vi "Digital Serial Acq Cfg Popup.vi"(8 "error in (no error)":errorcluster, 11 "config file in":path caption="Configuration File") -> (0 "error out":errorcluster, 2 "digital serial input settings":T2={"number of channels"=0, "data justification"=enum."Left Justified", "endianness"=enum."LSB First", "channel length"=0, "bit depth"=0, "frame clock rate"=0.0, "bit clock edge sync"=enum."Falling", "master clock source"=enum."Internal", "master clock rate"=2.0, "Logic Level"=enum."3.3 V", "frame sync edge for channel 0"=enum."Rising", "Channel 0 Offset"=0}, 3 "config file out":path caption="Configuration File")   [LabVIEW 2022 SP3, in "Config Dialog.lvlib"]
uses:
  Config Dialog.lvlib
  controls/digital serial audio/digital serial input settings.ctl
  <vilib>/PDM Acquisition Toolkit/shared/controls/PCM Data Justification.ctl
  <vilib>/PDM Acquisition Toolkit/shared/controls/PCM Bit Endianness.ctl
  <vilib>/PDM Acquisition Toolkit/shared/controls/Digital Edge.ctl
  controls/master clock source.ctl
  <vilib>/PDM Acquisition Toolkit/host/Classes/Session/Controls/Logic Levels.ctl
  <vilib>/Utility/miscctls.llb/LVPointTypeDef.ctl
  <vilib>/PDM Acquisition Toolkit/shared/PDM Shared.lvlib
  <vilib>/PDM Acquisition Toolkit/host/Classes/Session/DecoderSession.lvclass
  input configuration file/input cfg file.lvlib
  input configuration file/digital serial/digital serial input cfg file.lvlib
panel:
  in  "master clock source":T1 caption="Master clock source"
  in  "channel 0 offset":u32=1
  in  "Save":bool
  in  "logic level":enum32{"3.3 V", "1.8 V", "1.2 V"}(ring) caption="Logic level"
  in  "master clock rate":dbl=12288000.0 caption="Master clock rate" format="%#_6pHz"
  out "Bit clock rate":dbl=3072000.0 format="%#_6pHz"
  in  "number of channels":u32=2 caption="Number of channels"
  in  "TDM":bool
  in  "RJ":bool
  in  "LJ":bool
  in  "I2S":bool
  in  "bit clock edge sync":enum32{"Rising", "Falling"}(ring)=enum."Falling" caption="Bit clock edge sync"
  in  "frame clock rate":dbl=48000.0 caption="Frame clock rate" format="%#_6pHz"
  in  "data justification":enum32{"Left Justified", "Right Justified"}(ring) caption="Data justification"
  in  "endianness":enum32{"MSB First", "LSB First"}(ring) caption="Endianness"
  in  "bit depth":u32=24 caption="Bit depth"
  in  "channel length":u32=32 caption="Channel length"
  in  "frame sync edge for channel 0":enum32{"Rising", "Falling"}(ring)=enum."Falling" caption="Frame sync edge for Channel 0"
  # "Audio Protocol"
  # "Clock Settings"
  # "Signal Level"
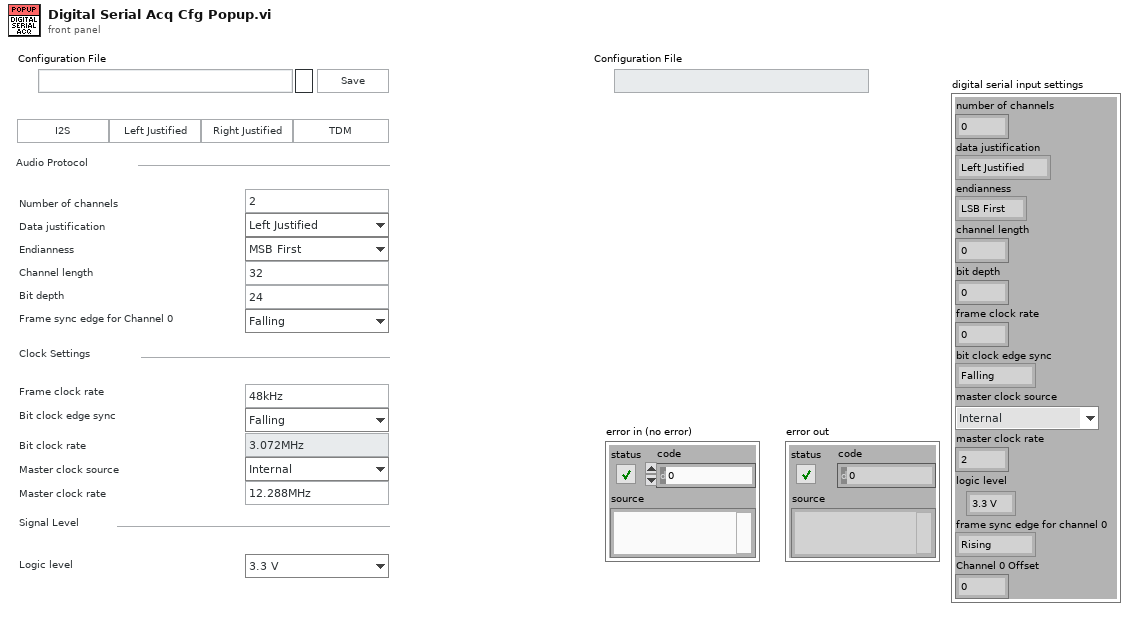
[diagram p1: front panel]
types:
  T1 = typedef "master clock source.ctl" = enum32{"Internal", "External"}
  T2 = typedef "digital serial input settings.ctl" = cluster{"number of channels":u32, "data justification":T3, "endianness":T4, "channel length":u32, "bit depth":u32, "frame clock rate":dbl, "bit clock edge sync":T5, "master clock source":T1, "master clock rate":dbl, "Logic Level":T6, "frame sync edge for channel 0":T5, "Channel 0 Offset":u32}
  T3 = typedef "PDM Shared.lvlib/PCM Data Justification.ctl" = enum16{"Left Justified", "Right Justified"}
  T4 = typedef "PDM Shared.lvlib/PCM Bit Endianness.ctl" = enum16{"MSB First", "LSB First"}
  T5 = typedef "PDM Shared.lvlib/Digital Edge.ctl" = enum8{"Rising", "Falling"}
  T6 = typedef "PDM Acquisition Class Library.lvlib/DecoderSession.lvclass/Logic Levels.ctl" = enum16{"3.3 V", "1.8 V", "1.2 V"}
  T7 = typedef "LVPointTypeDef.ctl" = cluster{"Horizontal":i16, "Vertical":i16}
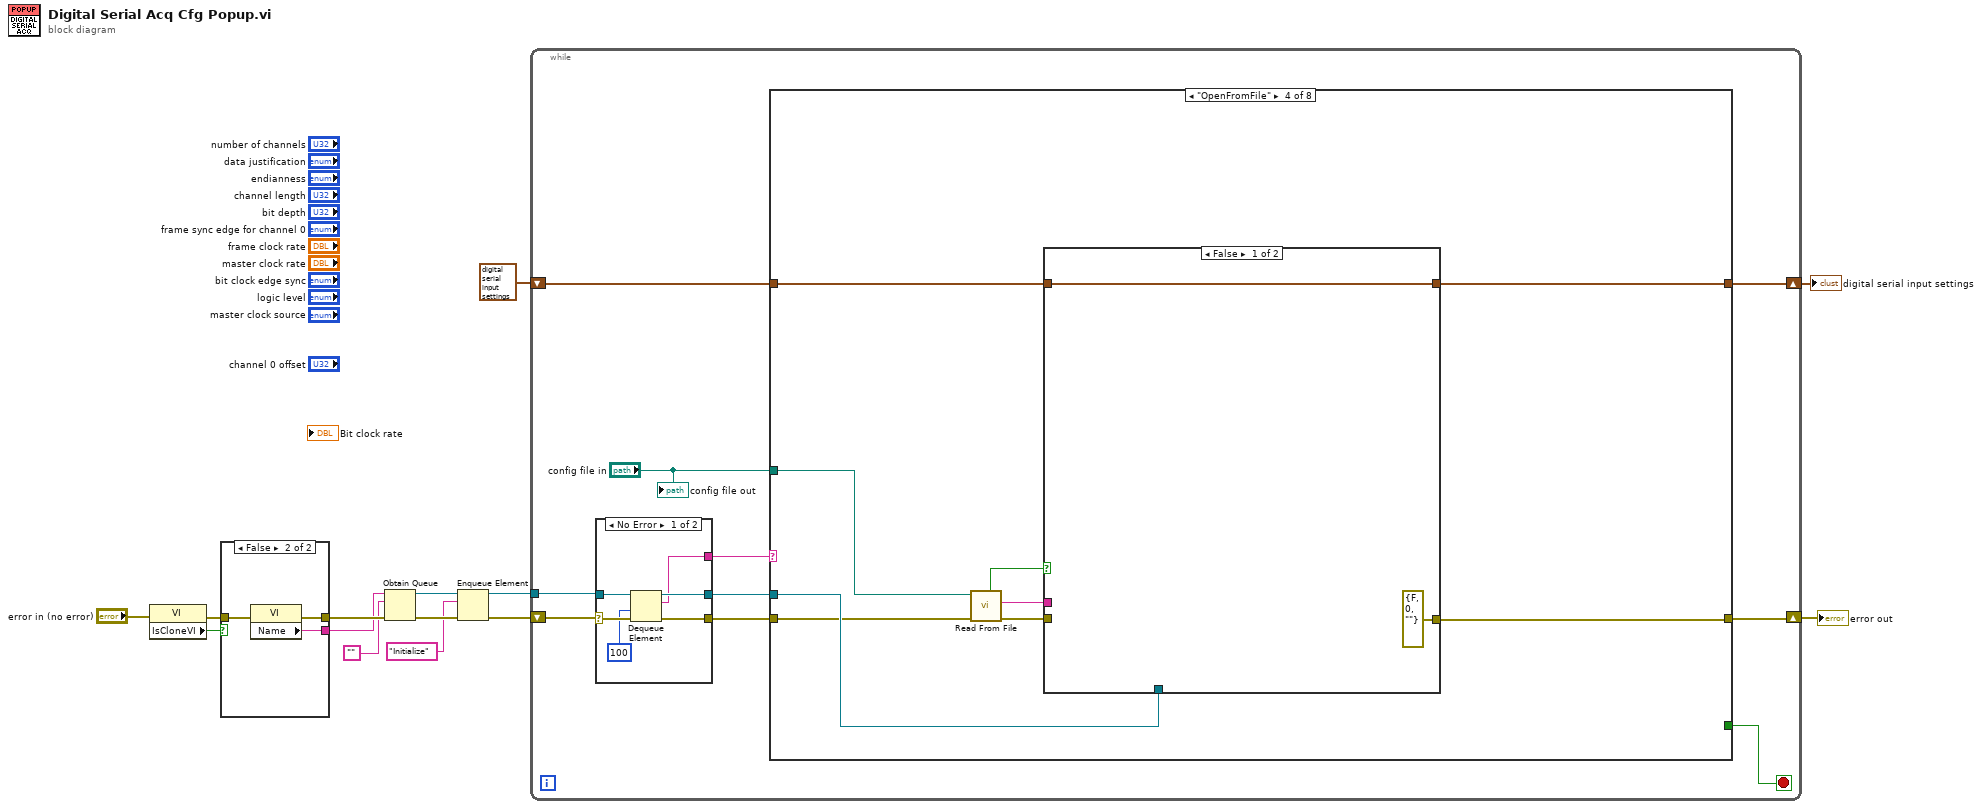
[diagram p0: block diagram]
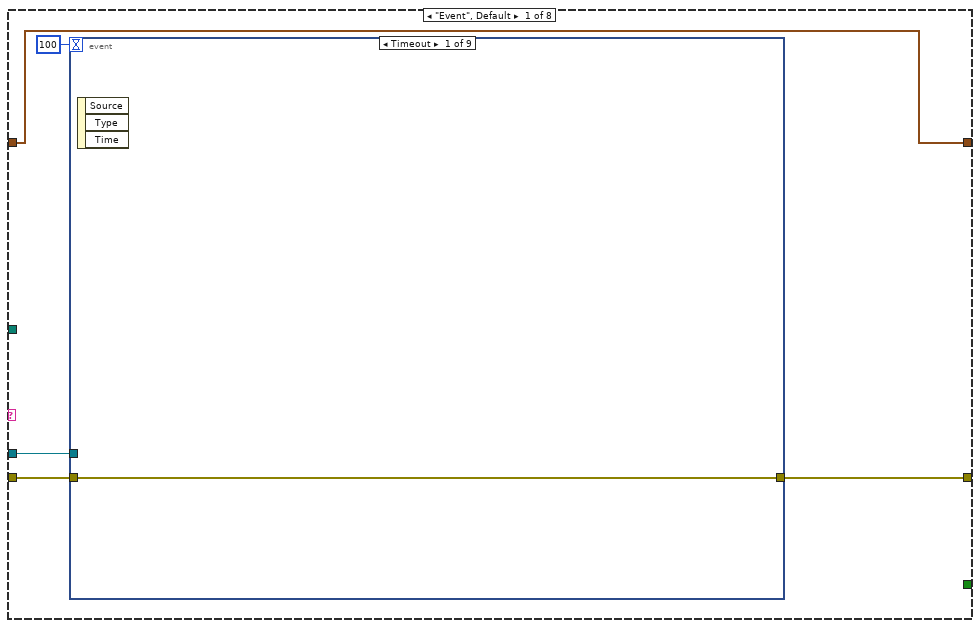
[diagram p2: hidden frame]
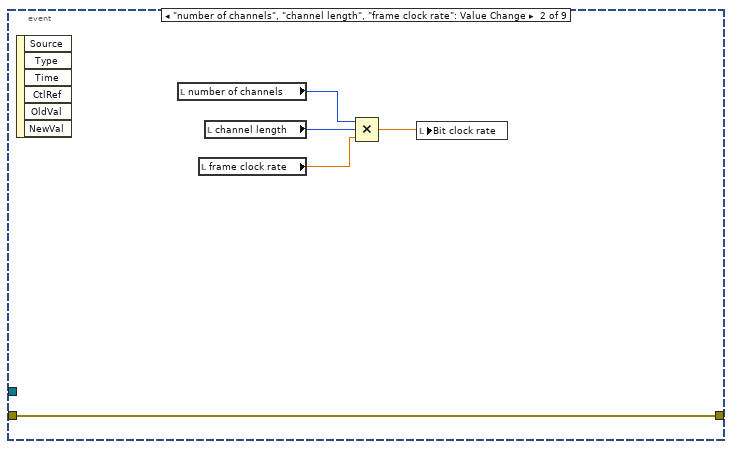
[diagram p3: hidden frame]
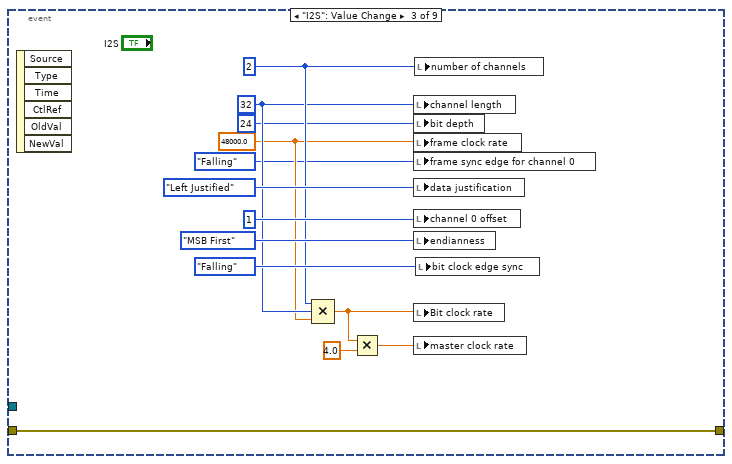
[diagram p4: hidden frame]
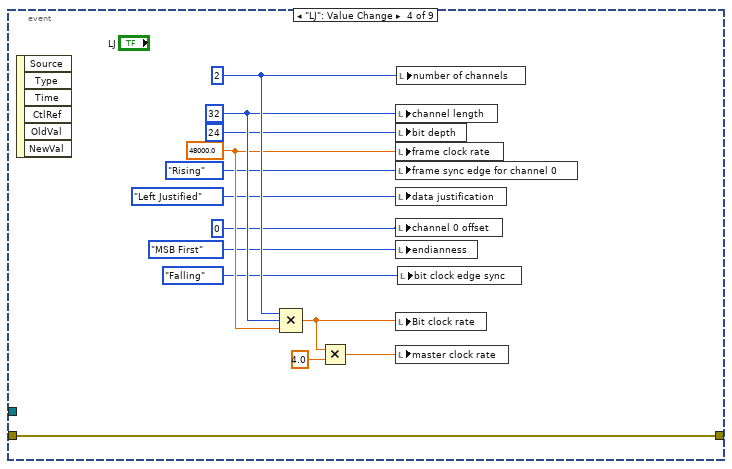
[diagram p5: hidden frame]
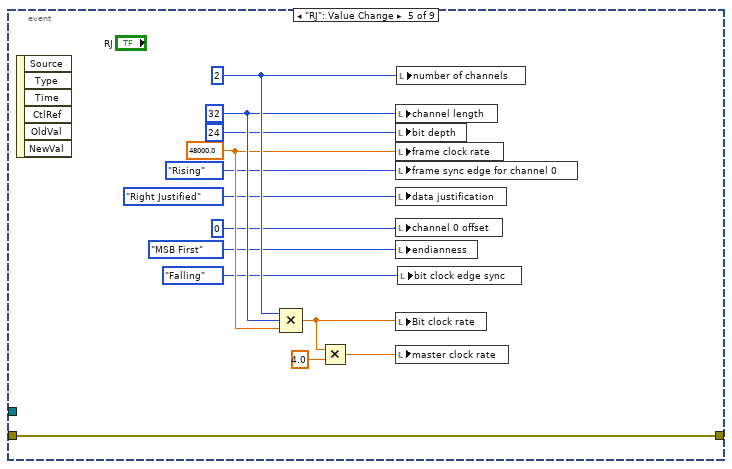
[diagram p6: hidden frame]
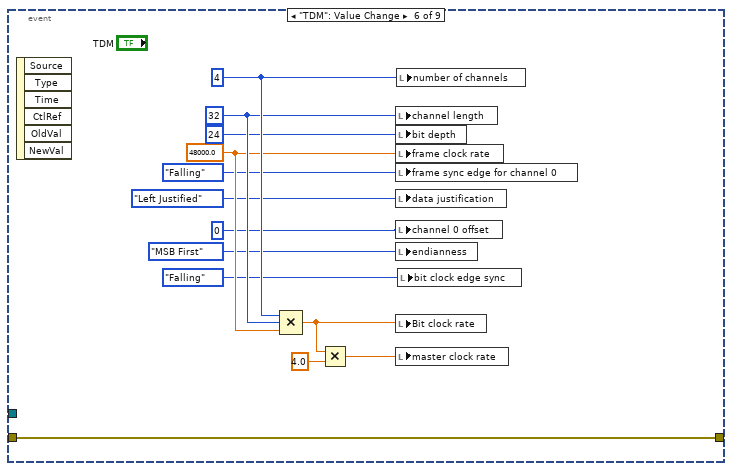
[diagram p7: hidden frame]
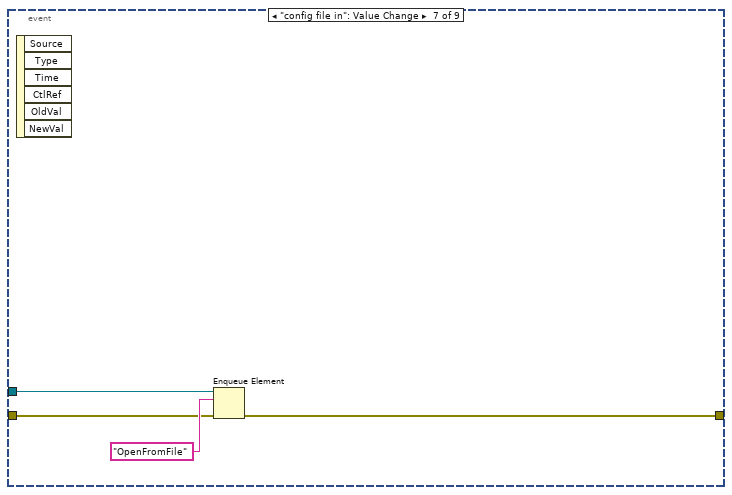
[diagram p8: hidden frame]
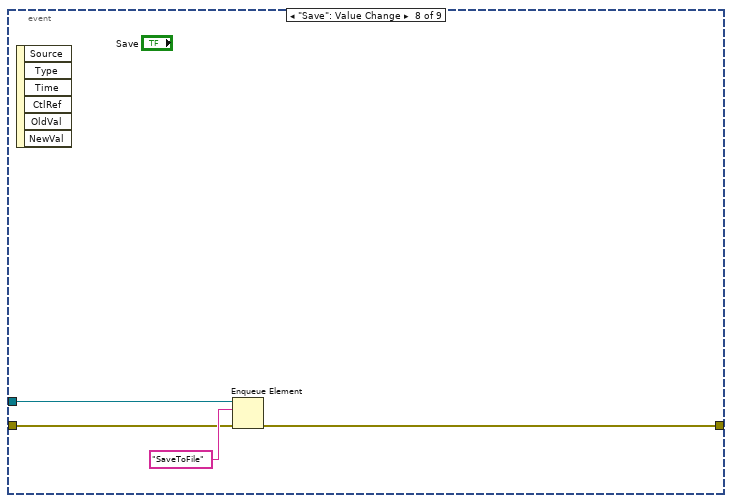
[diagram p9: hidden frame]
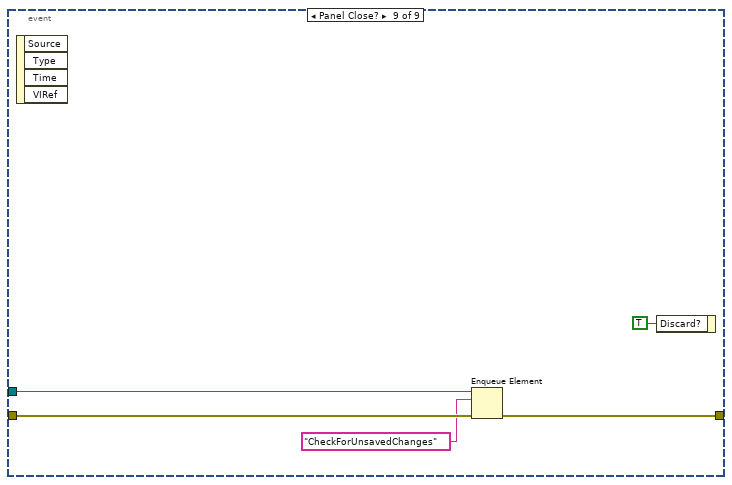
[diagram p10: hidden frame]
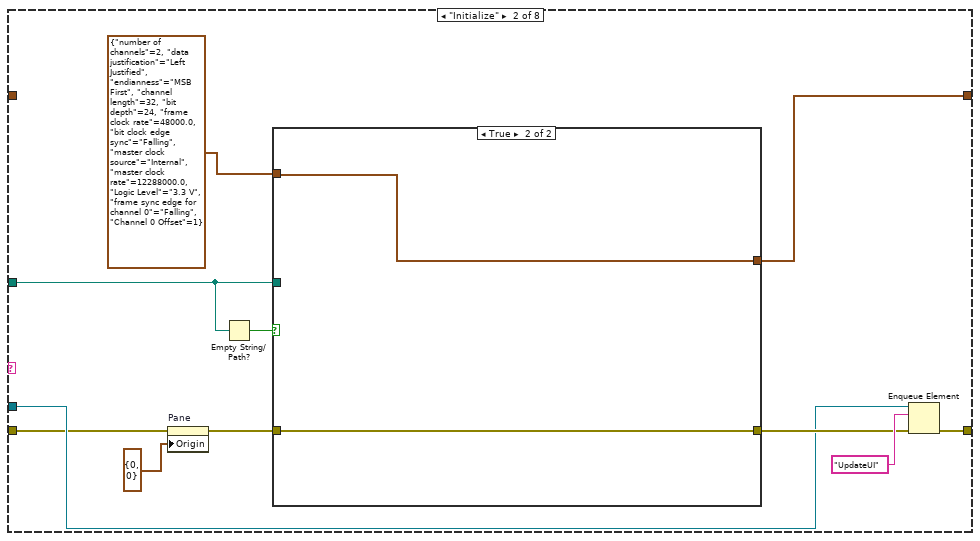
[diagram p11: hidden frame]
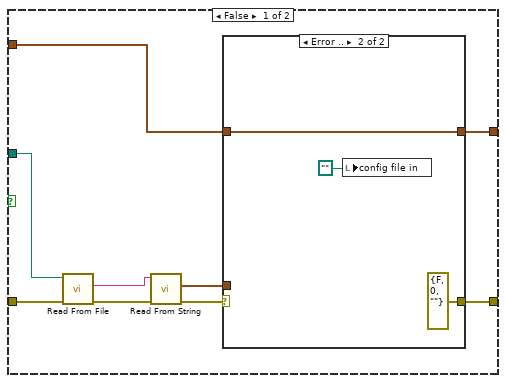
[diagram p12: hidden frame]
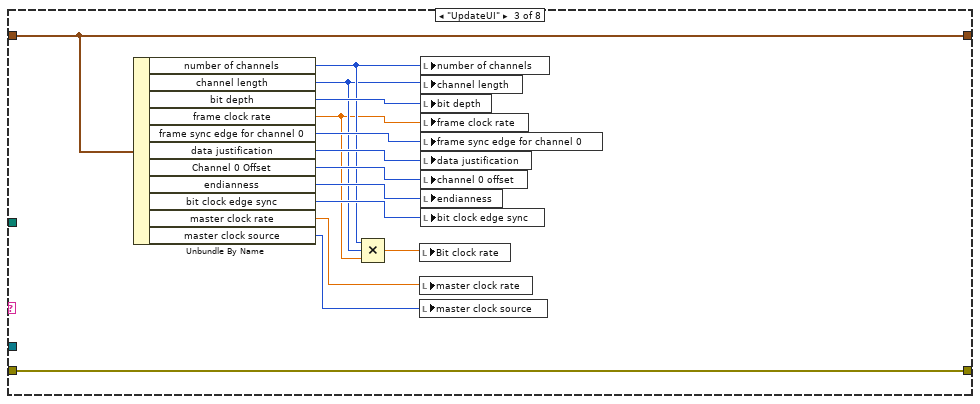
[diagram p14: hidden frame]
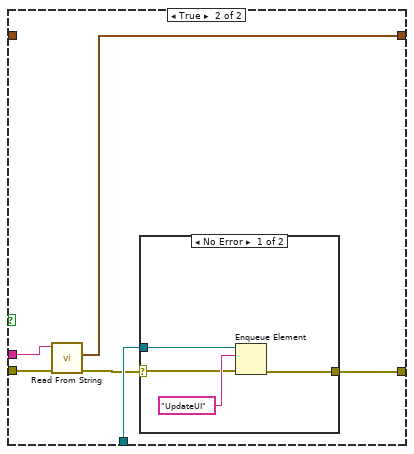
[diagram p15: hidden frame]
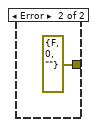
[diagram p16: hidden frame]
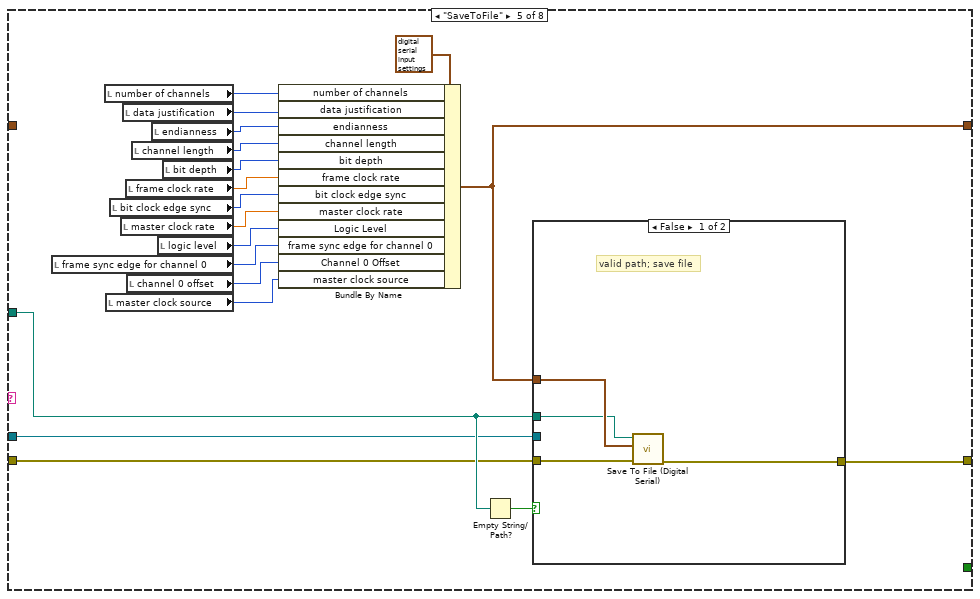
[diagram p17: hidden frame]
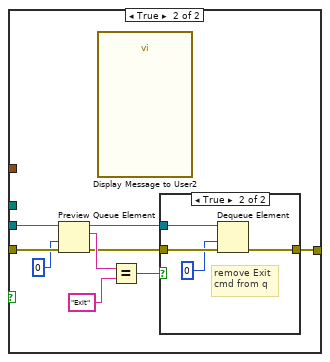
[diagram p18: hidden frame]
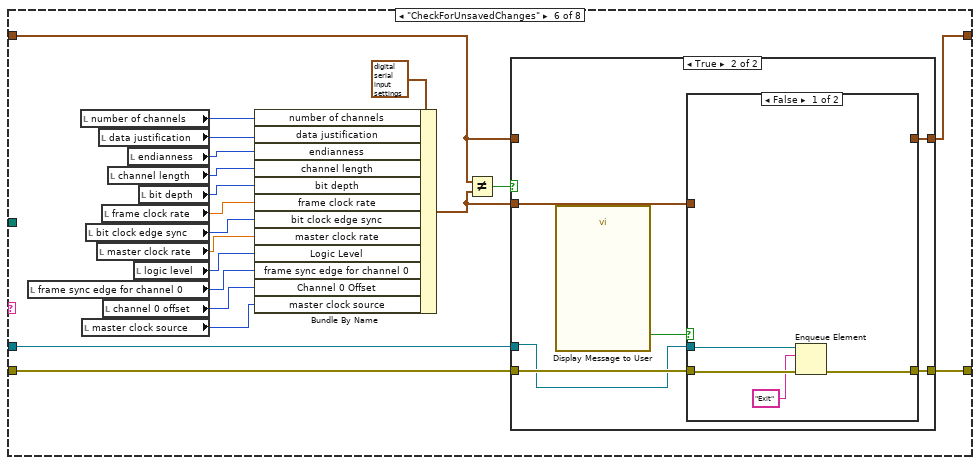
[diagram p20: hidden frame]
diagram:
  n1 = property class="VI"(error in="error in (no error)") -> (error out=w7:errorcluster, "IsCloneVI"=w8:bool)  [unwired: 1 in, 1 out]
  n2 = case shown="False" w8 {
    tunnel: [w17 w20] -> w14
    tunnel: [w16 w19] -> w13
    tunnel: w7 -> [w15 w18]
    frame True {
      n3 = property class="VI"(error in=w15) -> (error out=w17:errorcluster, "Clone Name"=w16:string)  [unwired: 1 in, 1 out]
    }
    frame False {
      n4 = property class="VI"(error in=w18) -> (error out=w20:errorcluster, "Name"=w19:string)  [unwired: 1 in, 1 out]
    }
  }
  n5 = Obtain Queue(name (unnamed)=w13, element data type="", error in (no error)=w14) -> (queue out=w11:refnum<queue>, error out=w12:errorcluster)  [unwired: 2 in, 1 out]
  n6 = Enqueue Element(queue=w11, element="Initialize", error in (no error)=w12) -> (queue out=w5:refnum<queue>, error out=w6:errorcluster)  [unwired: 1 in, 1 out]
  n7 = while {
    tunnel: w5 -> [w29]
    shift-right: [w25] -> w3
    shift-left: w6 -> [w30]
    shift-right: [w22] -> w1
    shift-left: T2 {"number of channels"=0, "data justification"=enum."Left Justified", "endianness"=enum."LSB First", "channel length"=0, "bit depth"=0, "frame clock rate"=0.0, "bit clock edge sync"=enum."Falling", "master clock source"=enum."Internal", "master clock rate"=2.0, "Logic Level"=enum."3.3 V", "frame sync edge for channel 0"=enum."Rising", "Channel 0 Offset"=0} ("digital serial input settings") -> [w23]
    stop <- w24 stop-if-true
    n8 = case shown="No Error" w30 {
      selector: w30 -> [w265 w268]
      tunnel: [w264 w268] -> w26
      tunnel: w29 -> [w263 w267]
      tunnel: [w262 w267] -> w27
      tunnel: [w261 "Handle Error"] -> w28
      frame No Error {
        n9 = Dequeue Element(queue=w263, timeout in ms (-1)=100, error in (no error)=w265) -> (queue out=w262:refnum<queue>, element=w261:string, error out=w264:errorcluster)  [unwired: 1 out]
      }
      frame Error {
      }
    }
    n10 = case shown="\"OpenFromFile\"" w28 {
      tunnel: w27 -> [w33 w112 _ w156 w171 w210 _ w255]
      tunnel: w26 -> [w34 w110 w147 w153 w173 w213 _ w256]
      tunnel: [w32 w113 w147 w155 w176 w212 errorcluster {"status"=FALSE, "code"=0, "source"=""} ("error out") w253] -> w25
      tunnel: [_ _ _ _ _ _ _ TRUE] -> w24
      tunnel: w23 -> [w31 _ w146 w151 _ w208 w251 w252]
      tunnel: [w31 w107 w146 w150 w175 w211 w251 w252] -> w22
      tunnel: "config file in" -> [_ w116 _ w154 w174 _ _ _]
      frame "Event", Default {
        n11 = event shown="[0] Timeout" {
          selector: _ -> [_ _ _ _ _ _ _ _ _]
          dyn-events: _ -> [_ _ _ _ _ _ _ _ _]
          timeout: 100 -> [_ _ _ _ _ _ _ _ _]
          tunnel: w34 -> [w36 w37 w42 w55 w68 w81 w96 w100 w105]
          tunnel: w33 -> [_ _ _ _ _ _ w95 w99 w104]
          tunnel: [w36 w37 w42 w55 w68 w81 w94 w98 w103] -> w32
          event Timeout {
            n12 = event-data() -> ()  [unwired: 1 in, 3 out]
          }
          event "number of channels", "channel length", "frame clock rate": Value Change {
            n13 = event-data() -> ()  [unwired: 1 in, 6 out]
            n14 = local read "number of channels"() -> (w39:u32)
            n15 = local read "frame clock rate"() -> (w38:dbl)
            n16 = local read "channel length"() -> (w40:u32)
            n17 = Compound Arithmetic op=MULTIPLY(w39, w40, w38) -> (w41:dbl)
            n18 = local write "Bit clock rate"(w41) -> ()
          }
          event "I2S": Value Change {
            w45 = 48000.0 ("Frame Clock Rate")
            w46 = u32 32 ("Channel Length")
            w47 = u32 2 ("Number of Channels")
            n19 = event-data() -> ()  [unwired: 1 in, 6 out]
            n20 = Compound Arithmetic op=MULTIPLY(w47, w46, w45) -> (w53:dbl)
            n21 = Multiply(x=w53, y=4.0) -> (x*y=w52:dbl)
            n22 = local write "channel length"(w46) -> ()
            n23 = local write "bit depth"(u32 24 ("Bit Depth")) -> ()
            n24 = local write "frame clock rate"(w45) -> ()
            n25 = local write "frame sync edge for channel 0"(enum32{"Rising", "Falling"}."Falling" ("bit clock edge sync")) -> ()
            n26 = local write "data justification"(enum32{"Left Justified", "Right Justified"}."Left Justified" ("data justification")) -> ()
            n27 = local write "channel 0 offset"(u32 1 ("Channel 0 Offset")) -> ()
            n28 = local write "endianness"(enum32{"MSB First", "LSB First"}."MSB First" ("endianness")) -> ()
            n29 = local write "Bit clock rate"(w53) -> ()
            n30 = local write "master clock rate"(w52) -> ()
            n31 = local write "number of channels"(w47) -> ()
            n32 = local write "bit clock edge sync"(enum32{"Rising", "Falling"}."Falling" ("frame sync edge for channel 0")) -> ()
          }
          event "LJ": Value Change {
            w63 = 48000.0 ("Frame Clock Rate")
            w65 = u32 32 ("Channel Length")
            w66 = u32 2 ("Number of Channels")
            n33 = event-data() -> ()  [unwired: 1 in, 6 out]
            n34 = Compound Arithmetic op=MULTIPLY(w66, w65, w63) -> (w57:dbl)
            n35 = Multiply(x=w57, y=4.0) -> (x*y=w56:dbl)
            n36 = local write "channel length"(w65) -> ()
            n37 = local write "bit depth"(u32 24 ("Bit Depth")) -> ()
            n38 = local write "frame clock rate"(w63) -> ()
            n39 = local write "frame sync edge for channel 0"(enum32{"Rising", "Falling"}."Rising" ("bit clock edge sync")) -> ()
            n40 = local write "data justification"(enum32{"Left Justified", "Right Justified"}."Left Justified" ("data justification")) -> ()
            n41 = local write "channel 0 offset"(u32 0 ("Channel 0 Offset")) -> ()
            n42 = local write "endianness"(enum32{"MSB First", "LSB First"}."MSB First" ("endianness")) -> ()
            n43 = local write "Bit clock rate"(w57) -> ()
            n44 = local write "master clock rate"(w56) -> ()
            n45 = local write "number of channels"(w66) -> ()
            n46 = local write "bit clock edge sync"(enum32{"Rising", "Falling"}."Falling" ("frame sync edge for channel 0")) -> ()
          }
          event "RJ": Value Change {
            w76 = 48000.0 ("Frame Clock Rate")
            w78 = u32 32 ("Channel Length")
            w79 = u32 2 ("Number of Channels")
            n47 = event-data() -> ()  [unwired: 1 in, 6 out]
            n48 = Compound Arithmetic op=MULTIPLY(w79, w78, w76) -> (w70:dbl)
            n49 = Multiply(x=w70, y=4.0) -> (x*y=w69:dbl)
            n50 = local write "channel length"(w78) -> ()
            n51 = local write "bit depth"(u32 24 ("Bit Depth")) -> ()
            n52 = local write "frame clock rate"(w76) -> ()
            n53 = local write "frame sync edge for channel 0"(enum32{"Rising", "Falling"}."Rising" ("bit clock edge sync")) -> ()
            n54 = local write "data justification"(enum32{"Left Justified", "Right Justified"}."Right Justified" ("data justification")) -> ()
            n55 = local write "channel 0 offset"(u32 0 ("Channel 0 Offset")) -> ()
            n56 = local write "endianness"(enum32{"MSB First", "LSB First"}."MSB First" ("endianness")) -> ()
            n57 = local write "Bit clock rate"(w70) -> ()
            n58 = local write "master clock rate"(w69) -> ()
            n59 = local write "number of channels"(w79) -> ()
            n60 = local write "bit clock edge sync"(enum32{"Rising", "Falling"}."Falling" ("frame sync edge for channel 0")) -> ()
          }
          event "TDM": Value Change {
            w89 = 48000.0 ("Frame Clock Rate")
            w91 = u32 32 ("Channel Length")
            w92 = u32 4 ("Number of Channels")
            n61 = event-data() -> ()  [unwired: 1 in, 6 out]
            n62 = Compound Arithmetic op=MULTIPLY(w92, w91, w89) -> (w83:dbl)
            n63 = Multiply(x=w83, y=4.0) -> (x*y=w82:dbl)
            n64 = local write "channel length"(w91) -> ()
            n65 = local write "bit depth"(u32 24 ("Bit Depth")) -> ()
            n66 = local write "frame clock rate"(w89) -> ()
            n67 = local write "frame sync edge for channel 0"(enum32{"Rising", "Falling"}."Falling" ("bit clock edge sync")) -> ()
            n68 = local write "data justification"(enum32{"Left Justified", "Right Justified"}."Left Justified" ("data justification")) -> ()
            n69 = local write "channel 0 offset"(u32 0 ("Channel 0 Offset")) -> ()
            n70 = local write "endianness"(enum32{"MSB First", "LSB First"}."MSB First" ("endianness")) -> ()
            n71 = local write "Bit clock rate"(w83) -> ()
            n72 = local write "master clock rate"(w82) -> ()
            n73 = local write "number of channels"(w92) -> ()
            n74 = local write "bit clock edge sync"(enum32{"Rising", "Falling"}."Falling" ("frame sync edge for channel 0")) -> ()
          }
          event "config file in": Value Change {
            n75 = event-data() -> ()  [unwired: 1 in, 6 out]
            n76 = Enqueue Element(queue=w95, element="OpenFromFile", error in (no error)=w96) -> (error out=w94:errorcluster)  [unwired: 1 in, 2 out]
          }
          event "Save": Value Change {
            n77 = event-data() -> ()  [unwired: 1 in, 6 out]
            n78 = Enqueue Element(queue=w99, element="SaveToFile", error in (no error)=w100) -> (error out=w98:errorcluster)  [unwired: 1 in, 2 out]
          }
          event Panel Close? {
            n79 = event-data() -> ()  [unwired: 1 in, 4 out]
            n80 = Enqueue Element(queue=w104, element="CheckForUnsavedChanges", error in (no error)=w105) -> (error out=w103:errorcluster)  [unwired: 1 in, 2 out]
            n81 = event-data("Discard?"=TRUE) -> ()  [unwired: 1 in, 1 out]
          }
        }
      }
      frame "Initialize" {
        n82 = property on="Pane" class="Pane"(error in=w110, "Origin"=T7 {"Horizontal"=0, "Vertical"=0}) -> (error out=w109:errorcluster)  [unwired: 1 in, 1 out]
        n83 = Empty String/Path?(string/path=w116) -> (empty?=w117:bool)
        n84 = case shown="True" w117 {
          tunnel: w109 -> [w121 w133]
          tunnel: w116 -> [w120 _]
          tunnel: [w125 w132] -> w107
          tunnel: [w126 w133] -> w114
          tunnel: T2 {"number of channels"=2, "data justification"=enum."Left Justified", "endianness"=enum."MSB First", "channel length"=32, "bit depth"=24, "frame clock rate"=48000.0, "bit clock edge sync"=enum."Falling", "master clock source"=enum."Internal", "master clock rate"=12288000.0, "Logic Level"=enum."3.3 V", "frame sync edge for channel 0"=enum."Falling", "Channel 0 Offset"=1} ("digital serial input settings") -> [w124 w132]
          frame False {
            n85 = call "Read From File.vi"("error in (no error)"=w121, "file path"=w120) -> ("error out"=w123:errorcluster, "input cfg JSON"=w122:string)  [unwired: 6 in, 2 out]
            n86 = call "Read From String.vi"("error in (no error)"=w123, "JSON string"=w122) -> ("error out"=w118:errorcluster, "digital serial input settings"=w119:T2)  [unwired: 8 in]
            n87 = case shown="Error .." w118 {
              selector: w118 -> [w128 _]
              tunnel: [w128 errorcluster {"status"=FALSE, "code"=0, "source"=""} ("error IO")] -> w126
              tunnel: w119 -> [w127 _]
              tunnel: [w127 w131] -> w125
              tunnel: w124 -> [_ w131]
              frame No Error {
              }
              frame Error {
                n88 = local write "config file in"(path "") -> ()
              }
            }
          }
          frame True {
          }
        }
        n89 = Enqueue Element(queue=w112, element="UpdateUI", error in (no error)=w114) -> (error out=w113:errorcluster)  [unwired: 1 in, 2 out]
      }
      frame "UpdateUI" {
        n90 = Unbundle By Name(w146) -> ("number of channels"=w139:u32, "channel length"=w138:u32, "bit depth"=w145:u32, "frame clock rate"=w137:dbl, "frame sync edge for channel 0"=w144:T5, "data justification"=w143:T3, "Channel 0 Offset"=w142:u32, "endianness"=w141:T4, "bit clock edge sync"=w140:T5, "master clock rate"=w135:dbl, "master clock source"=w134:T1)
        n91 = Compound Arithmetic op=MULTIPLY(w139, w138, w137) -> (w136:dbl)
        n92 = local write "Bit clock rate"(w136) -> ()
        n93 = local write "master clock rate"(w135) -> ()
        n94 = local write "master clock source"(w134) -> ()
        n95 = local write "number of channels"(w139) -> ()
        n96 = local write "channel length"(w138) -> ()
        n97 = local write "bit depth"(w145) -> ()
        n98 = local write "frame clock rate"(w137) -> ()
        n99 = local write "frame sync edge for channel 0"(w144) -> ()
        n100 = local write "data justification"(w143) -> ()
        n101 = local write "channel 0 offset"(w142) -> ()
        n102 = local write "endianness"(w141) -> ()
        n103 = local write "bit clock edge sync"(w140) -> ()
      }
      frame "OpenFromFile" {
        n104 = call "Read From File.vi"("error in (no error)"=w153, "file path"=w154) -> ("error out"=w149:errorcluster, "input cfg JSON"=w148:string, "file exists?"=w152:bool)  [unwired: 6 in, 1 out]
        n105 = case shown="False" w152 {
          tunnel: w156 -> [_ w164]
          tunnel: [errorcluster {"status"=FALSE, "code"=0, "source"=""} ("error out") w163] -> w155
          tunnel: w149 -> [_ w162]
          tunnel: w151 -> [w158 _]
          tunnel: [w158 w160] -> w150
          tunnel: w148 -> [_ w159]
          frame False {
          }
          frame True {
            n106 = call "Read From String.vi"("error in (no error)"=w162, "JSON string"=w159) -> ("error out"=w161:errorcluster, "digital serial input settings"=w160:T2)  [unwired: 8 in]
            n107 = case shown="No Error" w161 {
              selector: w161 -> [w165 _]
              tunnel: w164 -> [w167 _]
              tunnel: [w166 errorcluster {"status"=FALSE, "code"=0, "source"=""} ("error out")] -> w163
              frame No Error {
                n108 = Enqueue Element(queue=w167, element="UpdateUI", error in (no error)=w165) -> (error out=w166:errorcluster)  [unwired: 1 in, 2 out]
              }
              frame Error {
              }
            }
          }
        }
      }
      frame "SaveToFile" {
        n109 = local read "frame sync edge for channel 0"() -> (w178:enum32{"Rising", "Falling"})
        n110 = local read "number of channels"() -> (w187:u32)
        n111 = local read "master clock source"() -> (w170:T1)
        n112 = local read "bit clock edge sync"() -> (w181:enum32{"Rising", "Falling"})
        n113 = local read "master clock rate"() -> (w180:dbl)
        n114 = local read "data justification"() -> (w186:enum32{"Left Justified", "Right Justified"})
        n115 = local read "frame clock rate"() -> (w182:dbl)
        n116 = local read "channel 0 offset"() -> (w177:u32)
        n117 = local read "channel length"() -> (w184:u32)
        n118 = local read "endianness"() -> (w185:enum32{"MSB First", "LSB First"})
        n119 = local read "logic level"() -> (w179:enum32{"3.3 V", "1.8 V", "1.2 V"})
        n120 = local read "bit depth"() -> (w183:u32)
        n121 = Bundle By Name(cluster=T2 {"number of channels"=0, "data justification"=enum."Left Justified", "endianness"=enum."LSB First", "channel length"=0, "bit depth"=0, "frame clock rate"=0.0, "bit clock edge sync"=enum."Falling", "master clock source"=enum."Internal", "master clock rate"=2.0, "Logic Level"=enum."3.3 V", "frame sync edge for channel 0"=enum."Rising", "Channel 0 Offset"=0} ("input cluster"), "number of channels"=w187, "data justification"=w186, "endianness"=w185, "channel length"=w184, "bit depth"=w183, "frame clock rate"=w182, "bit clock edge sync"=w181, "master clock rate"=w180, "Logic Level"=w179, "frame sync edge for channel 0"=w178, "Channel 0 Offset"=w177, "master clock source"=w170) -> (w175:T2)
        n122 = Empty String/Path?(string/path=w174) -> (empty?=w172:bool)
        n123 = case shown="False" w172 {
          tunnel: [w192 w194] -> w176
          tunnel: w175 -> [w191 _]
          tunnel: w174 -> [w190 _]
          tunnel: w173 -> [w189 w201]
          tunnel: w171 -> [_ w200]
          frame False {
            # "valid path; save file"
            n124 = call "Save To File (Digital Serial).vi"("error in (no error)"=w189, "digital serial input settings"=w191, "file path"=w190) -> ("error out"=w192:errorcluster)  [unwired: 8 in]
          }
          frame True {
            n125 = Preview Queue Element(queue=w200, timeout in ms (-1)=0, error in (no error)=w201) -> (queue out=w197:refnum<queue>, element=w199:string, error out=w195:errorcluster)  [unwired: 1 out]
            n126 = call "Display Message to User2"() -> ()  [unwired: 10 in, 2 out]
            n127 = Equal?(x=w199, y="Exit") -> (x = y?=w196:bool)
            n128 = case shown="True" w196 {
              tunnel: w197 -> [_ w206]
              tunnel: w195 -> [w202 w205]
              tunnel: [w202 w204] -> w194
              frame False {
              }
              frame True {
                # "remove Exit\ncmd from q"
                n129 = Dequeue Element(queue=w206, timeout in ms (-1)=0, error in (no error)=w205) -> (error out=w204:errorcluster)  [unwired: 3 out]
              }
            }
          }
        }
      }
      frame "CheckForUnsavedChanges" {
        n130 = local read "frame sync edge for channel 0"() -> (w217:enum32{"Rising", "Falling"})
        n131 = local read "number of channels"() -> (w226:u32)
        n132 = local read "master clock source"() -> (w207:T1)
        n133 = local read "bit clock edge sync"() -> (w220:enum32{"Rising", "Falling"})
        n134 = local read "master clock rate"() -> (w219:dbl)
        n135 = local read "data justification"() -> (w225:enum32{"Left Justified", "Right Justified"})
        n136 = local read "frame clock rate"() -> (w221:dbl)
        n137 = local read "channel 0 offset"() -> (w216:u32)
        n138 = local read "channel length"() -> (w223:u32)
        n139 = local read "endianness"() -> (w224:enum32{"MSB First", "LSB First"})
        n140 = local read "logic level"() -> (w218:enum32{"3.3 V", "1.8 V", "1.2 V"})
        n141 = local read "bit depth"() -> (w222:u32)
        n142 = Bundle By Name(cluster=T2 {"number of channels"=0, "data justification"=enum."Left Justified", "endianness"=enum."LSB First", "channel length"=0, "bit depth"=0, "frame clock rate"=0.0, "bit clock edge sync"=enum."Falling", "master clock source"=enum."Internal", "master clock rate"=2.0, "Logic Level"=enum."3.3 V", "frame sync edge for channel 0"=enum."Rising", "Channel 0 Offset"=0} ("input cluster"), "number of channels"=w226, "data justification"=w225, "endianness"=w224, "channel length"=w223, "bit depth"=w222, "frame clock rate"=w221, "bit clock edge sync"=w220, "master clock rate"=w219, "Logic Level"=w218, "frame sync edge for channel 0"=w217, "Channel 0 Offset"=w216, "master clock source"=w207) -> (w209:T2)
        n143 = Not Equal?(x=w208, y=w209) -> (x != y?=w214:bool)
        n144 = case shown="True" w214 {
          tunnel: w213 -> [w229 w237]
          tunnel: [w227 w233] -> w212
          tunnel: w209 -> [_ w235]
          tunnel: w208 -> [w231 _]
          tunnel: [w231 w234] -> w211
          tunnel: w210 -> [w228 w232]
          frame False {
            n145 = Enqueue Element(queue=w228, element="Exit", error in (no error)=w229) -> (error out=w227:errorcluster)  [unwired: 1 in, 2 out]
          }
          frame True {
            n146 = call "Display Message to User"() -> ("Yes"=w236:bool)  [unwired: 10 in, 1 out]
            n147 = case shown="False" w236 {
              tunnel: w237 -> [w241 w248]
              tunnel: w235 -> [_ w247]
              tunnel: [_ w247] -> w234
              tunnel: [w239 w243] -> w233
              tunnel: w232 -> [w240 w242]
              frame False {
                n148 = Enqueue Element(queue=w240, element="Exit", error in (no error)=w241) -> (error out=w239:errorcluster)  [unwired: 1 in, 2 out]
              }
              frame True {
                n149 = Enqueue Element(queue=w242, element="SaveToFile", error in (no error)=w248) -> (queue out=w244:refnum<queue>, error out=w245:errorcluster)  [unwired: 1 in, 1 out]
                n150 = Enqueue Element(queue=w244, element="Exit", error in (no error)=w245) -> (error out=w243:errorcluster)  [unwired: 1 in, 2 out]
              }
            }
          }
        }
      }
      frame "Handle Error" {
      }
      frame "Exit" {
        n151 = Flush Queue(queue=w255, error in (no error)=w256) -> (queue out=w259:refnum<queue>, error out=w258:errorcluster)  [unwired: 1 out]
        n152 = Release Queue(queue=w259, force destroy? (F)=TRUE, error in (no error)=w258) -> (error out=w253:errorcluster)  [unwired: 2 out]
      }
    }
    "config file out" <- "config file in"
  }
  "error out" <- w3
  "digital serial input settings" <- w1
